vi "FILTERS_AI.vi"(9 "sampling freq: fs":dbl=1.0 format="%0.2f", 10 "Array":T1(array[cluster]) {"low cutoff freq: fl" format="%0.4f"}, 11 "data in":waveform(dbl)[](array[waveform])) -> (3 "filtered":waveform(dbl)[](array[waveform]))   [LabVIEW 2016]
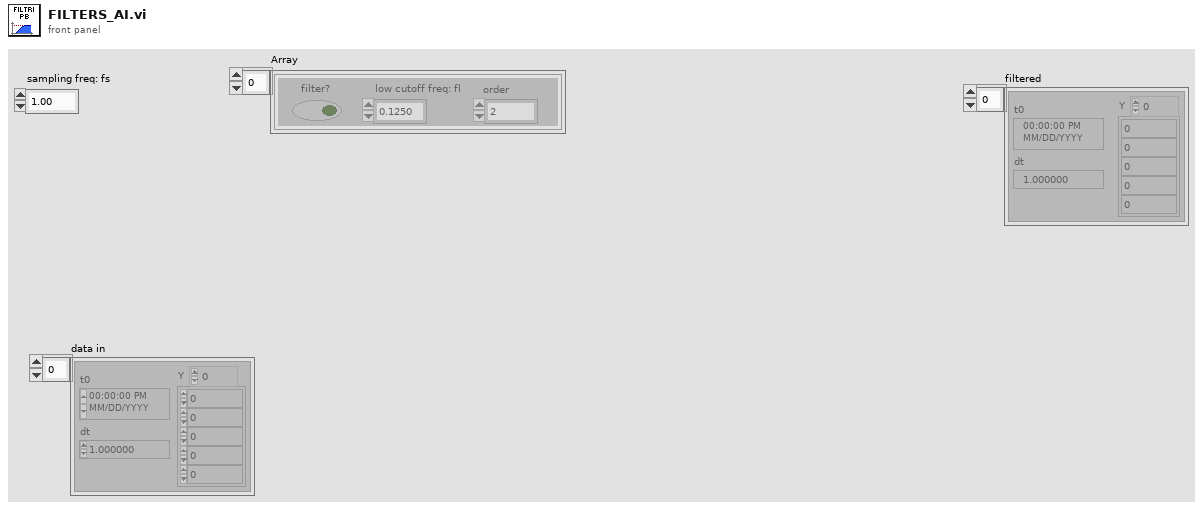
[diagram p1: front panel]
types:
  T1 = cluster{"filter?":bool, "low cutoff freq: fl":dbl, "order":i32}[]
  T2 = cluster{"filter?":bool, "low cutoff freq: fl":dbl, "order":i32}
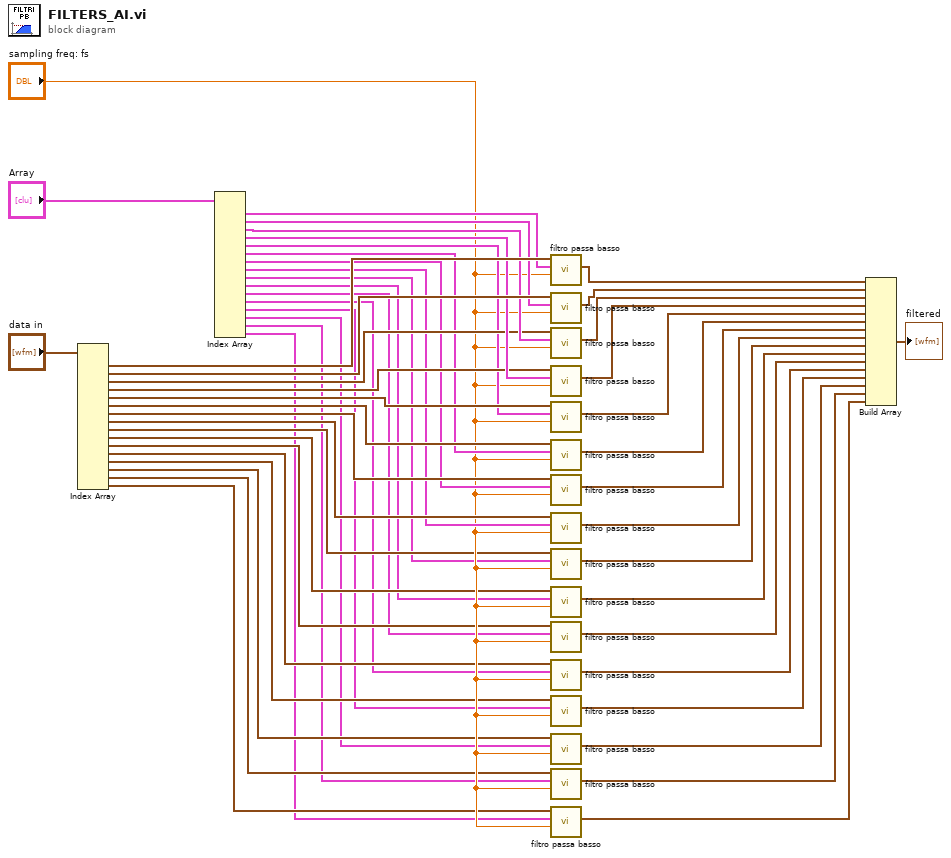
[diagram p0: block diagram]
diagram:
  n1 = Index Array(array="data in") -> (element #1=w52:waveform(dbl), element #2=w48:waveform(dbl), element #3=w44:waveform(dbl), element #4=w43:waveform(dbl), element #5=w42:waveform(dbl), element #6=w40:waveform(dbl), element #7=w38:waveform(dbl), element #8=w36:waveform(dbl), element #9=w33:waveform(dbl), element #10=w32:waveform(dbl), element #11=w31:waveform(dbl), element #12=w30:waveform(dbl), element #13=w29:waveform(dbl), element #14=w28:waveform(dbl), element #15=w27:waveform(dbl), element #16=w26:waveform(dbl))  [unwired: 16 in]
  n2 = Index Array(array="Array") -> (element #1=w49:T2, element #2=w47:T2, element #3=w46:T2, element #4=w45:T2, element #5=w41:T2, element #6=w39:T2, element #7=w37:T2, element #8=w35:T2, element #9=w25:T2, element #10=w24:T2, element #11=w23:T2, element #12=w22:T2, element #13=w21:T2, element #14=w20:T2, element #15=w19:T2, element #16=w18:T2)  [unwired: 16 in]
  n3 = call "filtro passa basso.vi"("sampling freq: fs"="sampling freq: fs", "Cluster"=w49, "Waveform"=w52) -> ("Waveform 2"=w17:waveform(dbl))  [unwired: 8 in]
  n4 = call "filtro passa basso.vi"("sampling freq: fs"="sampling freq: fs", "Cluster"=w47, "Waveform"=w48) -> ("Waveform 2"=w16:waveform(dbl))  [unwired: 8 in]
  n5 = call "filtro passa basso.vi"("sampling freq: fs"="sampling freq: fs", "Cluster"=w46, "Waveform"=w44) -> ("Waveform 2"=w15:waveform(dbl))  [unwired: 8 in]
  n6 = call "filtro passa basso.vi"("sampling freq: fs"="sampling freq: fs", "Cluster"=w45, "Waveform"=w43) -> ("Waveform 2"=w14:waveform(dbl))  [unwired: 8 in]
  n7 = call "filtro passa basso.vi"("sampling freq: fs"="sampling freq: fs", "Cluster"=w41, "Waveform"=w42) -> ("Waveform 2"=w13:waveform(dbl))  [unwired: 8 in]
  n8 = call "filtro passa basso.vi"("sampling freq: fs"="sampling freq: fs", "Cluster"=w39, "Waveform"=w40) -> ("Waveform 2"=w12:waveform(dbl))  [unwired: 8 in]
  n9 = call "filtro passa basso.vi"("sampling freq: fs"="sampling freq: fs", "Cluster"=w37, "Waveform"=w38) -> ("Waveform 2"=w11:waveform(dbl))  [unwired: 8 in]
  n10 = call "filtro passa basso.vi"("sampling freq: fs"="sampling freq: fs", "Cluster"=w35, "Waveform"=w36) -> ("Waveform 2"=w10:waveform(dbl))  [unwired: 8 in]
  n11 = call "filtro passa basso.vi"("sampling freq: fs"="sampling freq: fs", "Cluster"=w25, "Waveform"=w33) -> ("Waveform 2"=w9:waveform(dbl))  [unwired: 8 in]
  n12 = call "filtro passa basso.vi"("sampling freq: fs"="sampling freq: fs", "Cluster"=w24, "Waveform"=w32) -> ("Waveform 2"=w8:waveform(dbl))  [unwired: 8 in]
  n13 = call "filtro passa basso.vi"("sampling freq: fs"="sampling freq: fs", "Cluster"=w23, "Waveform"=w31) -> ("Waveform 2"=w7:waveform(dbl))  [unwired: 8 in]
  n14 = call "filtro passa basso.vi"("sampling freq: fs"="sampling freq: fs", "Cluster"=w22, "Waveform"=w30) -> ("Waveform 2"=w6:waveform(dbl))  [unwired: 8 in]
  n15 = call "filtro passa basso.vi"("sampling freq: fs"="sampling freq: fs", "Cluster"=w21, "Waveform"=w29) -> ("Waveform 2"=w5:waveform(dbl))  [unwired: 8 in]
  n16 = call "filtro passa basso.vi"("sampling freq: fs"="sampling freq: fs", "Cluster"=w20, "Waveform"=w28) -> ("Waveform 2"=w4:waveform(dbl))  [unwired: 8 in]
  n17 = call "filtro passa basso.vi"("sampling freq: fs"="sampling freq: fs", "Cluster"=w19, "Waveform"=w27) -> ("Waveform 2"=w3:waveform(dbl))  [unwired: 8 in]
  n18 = call "filtro passa basso.vi"("sampling freq: fs"="sampling freq: fs", "Cluster"=w18, "Waveform"=w26) -> ("Waveform 2"=w2:waveform(dbl))  [unwired: 8 in]
  n19 = Build Array(w17, w16, w15, w14, w13, w12, w11, w10, w9, w8, w7, w6, w5, w4, w3, w2) -> (→"filtered":waveform(dbl)[])
